vi "Prepare To Execute.vi"(0 "WriteCommand in":refnum<class "WriteCommand.lvclass">, 5 "error in (no error)":errorcluster) -> (14 "WriteCommand out":refnum<class "WriteCommand.lvclass">, 15 "Driver out":refnum<class "Driver.lvclass">, 16 "Executable":refnum<class "Executable.lvclass">, 19 "error out":errorcluster)   [LabVIEW 2023, in "HAF.lvlib" / "WriteCommand.lvclass"]
doc: "Makes the necessary preparations for executing the Command: initialising the Driver and the Driver Settings."
uses:
  WriteCommand.lvclass
  WriteCommand.lvclass/WriteCommand.ctl
  Executable/Executable.lvclass
  Driver/Driver.lvclass
  \\Mac\Home/Documents/LabVIEW Data/ProjectTemplates/Source/HAF/WriteCommand/WriteCommand.lvclass
  \\Mac\Home/Documents/LabVIEW Data/ProjectTemplates/Source/HAF/Executable/Executable.lvclass
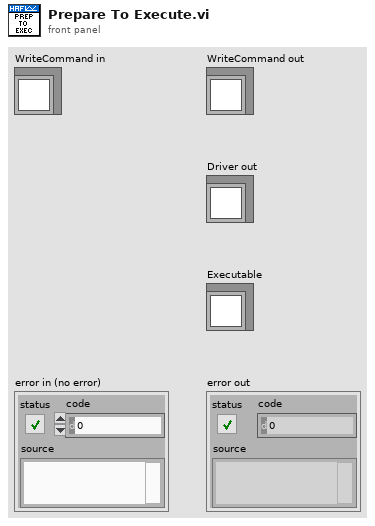
[diagram p1: front panel]
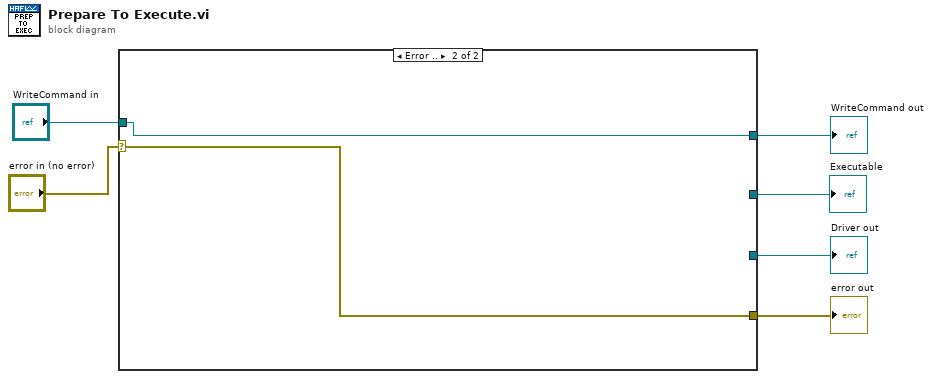
[diagram p0: block diagram]
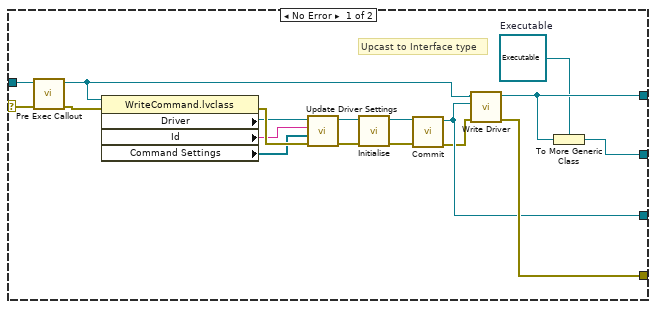
[diagram p2: hidden frame]
diagram:
  n1 = case shown="Error .." "error in (no error)" {
    selector: "error in (no error)" -> [w7 w25]
    tunnel: [w24 w26] -> w6
    tunnel: [w23 _] -> w5
    tunnel: [w21 w25] -> w4
    tunnel: [w20 _] -> w3
    tunnel: "WriteCommand in" -> [w8 w26]
    frame No Error {
      w22 = refnum<class "Executable.lvclass"> refnum  # Executable
      # "Upcast to Interface type"
      n2 = call-dynamic "Pre Exec Callout.vi"("error in (no error)"=w7, "WriteCommand in"=w8) -> ("error out"=w9:errorcluster, "WriteCommand out"=w18:refnum<class "WriteCommand.lvclass">)  [unwired: 8 in]
      n3 = property class="WriteCommand.lvclass"(reference=w18, error in=w9) -> (error out=w13:errorcluster, "Driver"=w10:refnum<class "Driver.lvclass">, "Id"=w11:string, "Command Settings"=w12:refnum<class "CommandSetting.lvclass">[])  [unwired: 1 out]
      n4 = call-dynamic "Update Driver Settings.vi"("error in (no error)"=w13, "Command Settings"=w12, "Command Id"=w11, "Driver in"=w10) -> ("error out"=w15:errorcluster, "Driver out"=w14:refnum<class "Driver.lvclass">)  [unwired: 4 in, 2 out]
      n5 = call-dynamic "Initialise.vi"("error in (no error)"=w15, "Driver in"=w14) -> ("error out"=w17:errorcluster, "Driver out"=w16:refnum<class "Driver.lvclass">)  [unwired: 8 in]
      n6 = call-dynamic "Commit.vi"("error in (no error)"=w17, "Driver in"=w16) -> ("error out"=w19:errorcluster, "Driver out"=w20:refnum<class "Driver.lvclass">)  [unwired: 8 in]
      n7 = call-dynamic "Write Driver.vi"("error in (no error)"=w19, "HAF:Driver.lvclass"=w20, "WriteCommand in"=w18) -> ("error out"=w21:errorcluster, "WriteCommand out"=w24:refnum<class "WriteCommand.lvclass">)  [unwired: 7 in]
      n8 = To More Generic Class(target class=w22, reference=w24) -> (generic class reference=w23:refnum<class "Executable.lvclass">)
    }
    frame Error {
    }
  }
  "WriteCommand out" <- w6
  "Executable" <- w5
  "error out" <- w4
  "Driver out" <- w3
